vi "Test Resampling.vi"() -> ()   [LabVIEW 2019, in "Instrument.Lockin.lvlib" / "Instrument.DAQ.lvclass"]
uses:
  Instrument.DAQ.lvclass
  <vilib>/measure/NI_MABase.lvlib
panel:
  out "Numeric":i32
  in  "stop":bool
  out "x-y":dbl
  in  "sampling info":cluster{"Fs":dbl, "#s":dbl}={"Fs"=1000.0, "#s"=1000.0}
  out "Waveform Graph":waveform(dbl)[](graph)
  in  "frequency":dbl[](array[numeric]) format="%0.2p"
  in  "output fs[Hz]":dbl=6500.0 format="%#_13g"
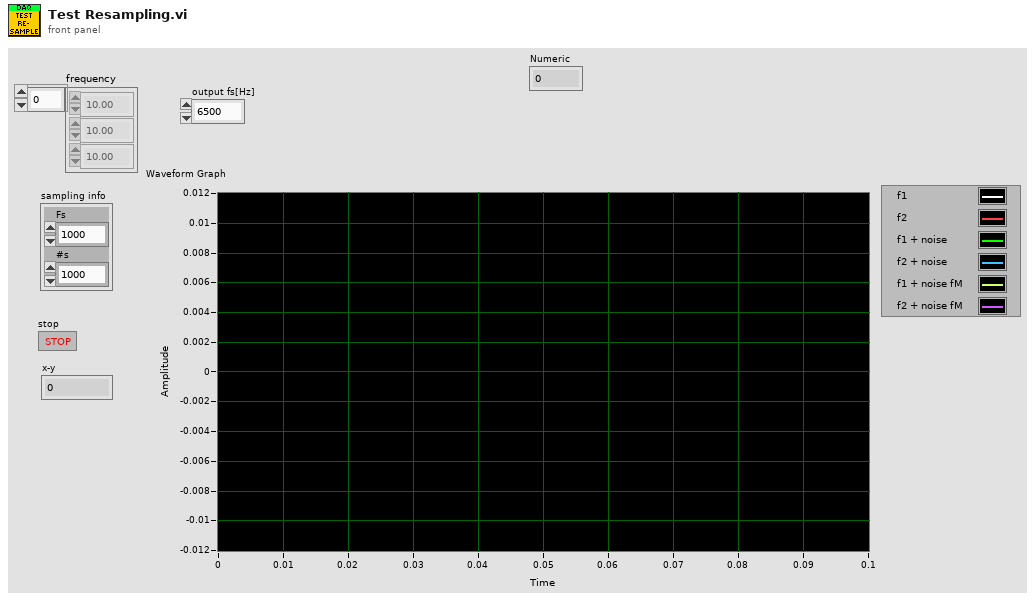
[diagram p1: front panel]
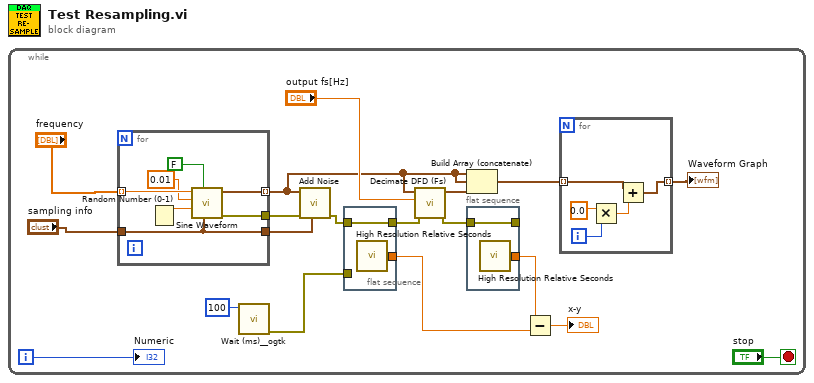
[diagram p0: block diagram]
diagram:
  n1 = while {
    i -> [w5]
    stop <- "stop" stop-if-true
    n2 = for {
      tunnel: [w35] -> w13 mode=indexing
      tunnel: "sampling info" -> [w34]
      tunnel: [w34] -> w18
      tunnel: [w33] -> w17
      tunnel: "frequency" -> [w32] mode=indexing
      n3 = Random Number (0-1)() -> (number: 0 to 1=w29:dbl)
      n4 = call <vilib>:"Sine Waveform.vi"("sampling info"=w34, "reset signal"=FALSE, "phase"=w29, "amplitude"=0.01, "frequency"=w32) -> ("error out"=w33:errorcluster, "signal out"=w35:waveform(dbl))  [unwired: 5 in]
    }
    n5 = call <userlib>:"Wait (ms)__ogtk.vi"("milliseconds to wait"=u32 100) -> ("error out"=w4:errorcluster)  [unwired: 9 in, 1 out]
    n6 = call "Add Noise.vi"("Sampling"=w18, "error in (no error)"=w17, "AI []"=w13) -> ("error out"=w12:errorcluster)  [unwired: 7 in, 1 out]
    n7 = flat-sequence {
      tunnel: w12 -> [w23]
      tunnel: [w23] -> w11
      tunnel: [w22] -> w8
      tunnel: w4 -> [_]
      frame #0 {
        n8 = call <vilib>:"High Resolution Relative Seconds.vi"() -> ("relative seconds"=w22:dbl)
      }
    }
    n9 = call "Decimate DFD (Fs).vi"("error in (no error)"=w11, "output fs[Hz]"="output fs[Hz]", "Waveforms in"=w13) -> ("error out"=w10:errorcluster, "waveforms out"=w16:waveform(dbl)[])  [unwired: 7 in]
    n10 = Build Array (concatenate)(w13, w13, w16) -> (w15:waveform(dbl)[])
    n11 = flat-sequence {
      tunnel: w10 -> [w21]
      tunnel: [w21] -> _
      tunnel: [w20] -> w9
      frame #0 {
        n12 = call <vilib>:"High Resolution Relative Seconds.vi"() -> ("relative seconds"=w20:dbl)
      }
    }
    n13 = Subtract(x=w9, y=w8) -> (x-y=→"x-y":dbl)
    n14 = for {
      tunnel: w15 -> [w25] mode=indexing
      tunnel: [w24] -> w14 mode=indexing
      i -> [w28]
      n15 = Multiply(x=0.0 ("amplitude"), y=w28) -> (x*y=w26:dbl)
      n16 = Add(x=w25, y=w26) -> (x+y=w24:waveform(dbl))
    }
    "Waveform Graph" <- w14
    "Numeric" <- w5
  }
